vi "Write SystemConfig.vi"(8 "error in (no error)":errorcluster, 10 "SystemConfig":T1, 11 "SystemConfiguration in":refnum<class "SystemConfiguration.lvclass">) -> (0 "error out":errorcluster, 3 "SystemConfiguration out":refnum<class "SystemConfiguration.lvclass">)   [LabVIEW 2019, in "SystemSetup.lvlib" / "SystemConfiguration.lvclass"]
uses:
  SystemConfiguration.lvclass
  SystemConfig.ctl
  SystemConfiguration.lvclass/SystemConfiguration.ctl
  SystemSetup.lvclass
panel:
  # "StationInfo"
  # "SaveDataPath"
  # "TestStand"
  # "CurrentImage"
  # "BarCodeScanner"
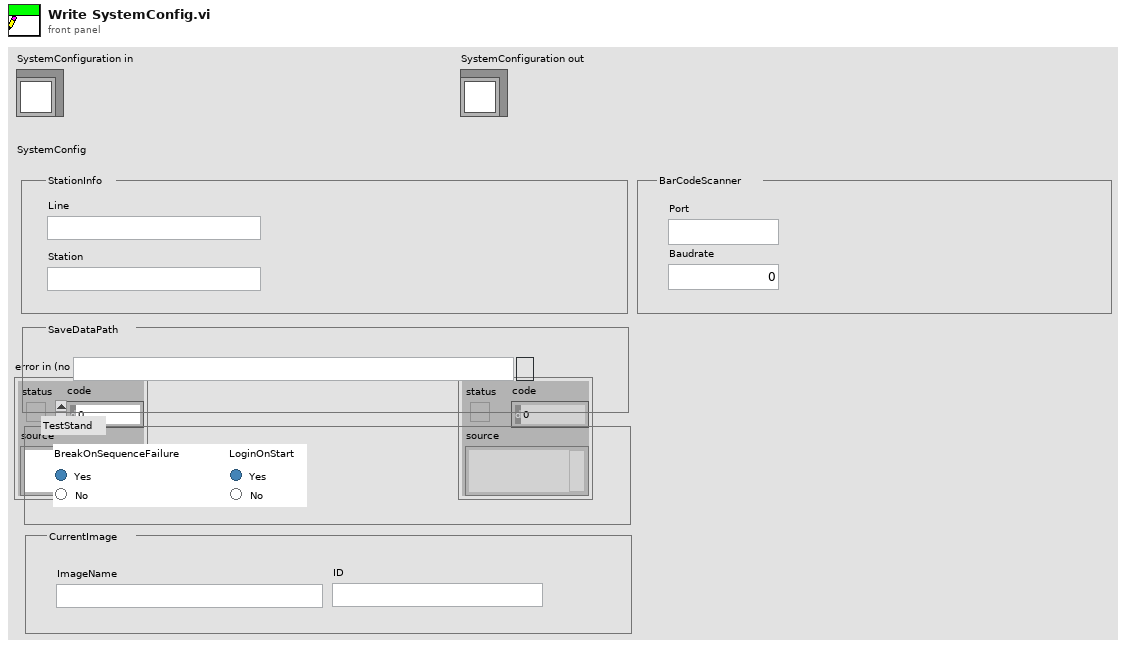
[diagram p1: front panel]
types:
  T1 = typedef "SystemSetup.lvlib/SystemSetup.lvclass/SystemConfig.ctl" = cluster{"StationInfo":cluster{"Line":string, "Station":string}, "SaveDataPath":cluster{"Path":path}, "TestStand":cluster{"BreakOnSequenceFailure":enum32{"Yes", "No"}, "LoginOnStart":enum32{"Yes", "No"}}, "CurrentImage":cluster{"ImageName":string, "ID":string}, "HardwareConfiguration":cluster{"BarCodeScanner":cluster{"Port":string, "Baudrate":i32}}}
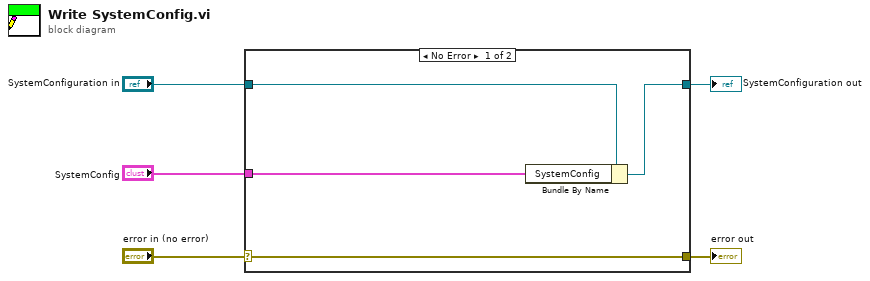
[diagram p0: block diagram]
diagram:
  n1 = case shown="No Error" "error in (no error)" {
    selector: "error in (no error)" -> [w9 w10]
    tunnel: [w9 w10] -> w4
    tunnel: [w7 w11] -> w2
    tunnel: "SystemConfiguration in" -> [w8 w11]
    tunnel: "SystemConfig" -> [w6 _]
    frame No Error {
      n2 = Bundle By Name(cluster=w8, "SystemConfig"=w6) -> (w7:refnum<class "SystemConfiguration.lvclass">)
    }
    frame Error {
    }
  }
  "error out" <- w4
  "SystemConfiguration out" <- w2
